vi "LVDeleteFile_Item_OnCommand.vi"(10 "Command ID":string, 11 "Object":T1) -> ()   [LabVIEW 2018]
uses:
  <resource>/Framework/Providers/API/ItemRef.ctl
panel:
  out "error out":errorcluster
  in  "error in":errorcluster
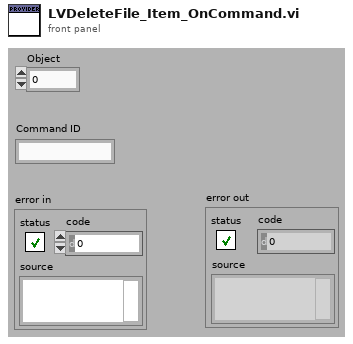
[diagram p1: front panel]
types:
  T1 = typedef "ItemRef.ctl" = u64
  T2 = enum16{"Left Button", "Center Button", "Right Button", "Window Close"}
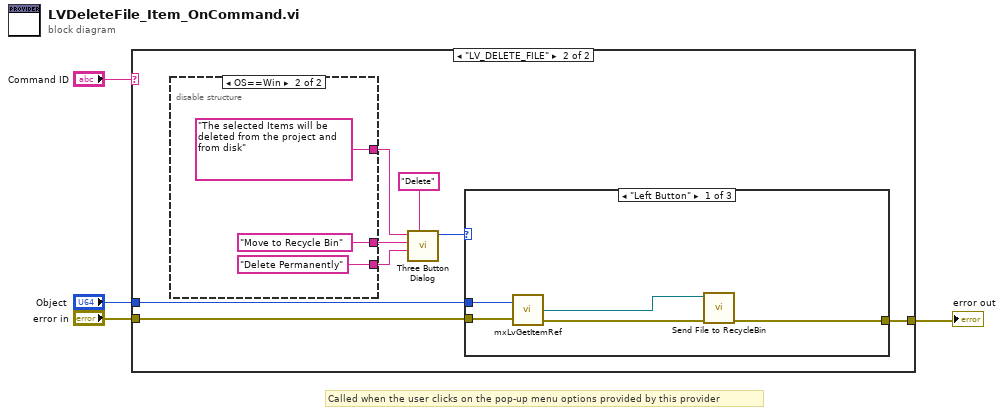
[diagram p0: block diagram]
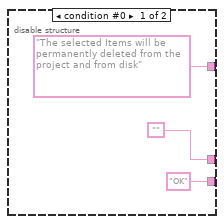
[diagram p3: hidden frame]
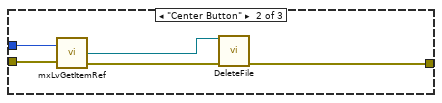
[diagram p4: hidden frame]
diagram:
  # "Called when the user clicks on the pop-up menu options provided by this provider"
  n1 = case shown="\"LV_DELETE_FILE\"" "Command ID" {
    tunnel: "error in" -> [w5 w13]
    tunnel: [w5 w12] -> w2
    tunnel: "Object" -> [_ w11]
    frame Default {
    }
    frame "LV_DELETE_FILE" {
      n2 = disable-structure shown="OS==Win" {
        disable-tunnel: ["The selected Items will be permanently deleted from the project and from disk" ("message") "The selected Items will be deleted from the project and from disk" ("message")] -> w10
        disable-tunnel: ["" "Move to Recycle Bin" ("message")] -> w8
        disable-tunnel: ["OK" ("message") "Delete Permanently" ("message")] -> w7
        frame condition #0 {
        }
        frame condition #1 (active) {
        }
      }
      n3 = call <vilib>:"Three Button Dialog.vi"("Window Title (\"\")"="Delete" ("Window Title (\"\")"), "Center Button Text (\"No\")"=w7, "Left Button Text (\"Yes\")"=w8, "message"=w10) -> ("Which Button?"=w9:T2)  [unwired: 7 in]
      n4 = case shown="\"Left Button\"" w9 {
        tunnel: w11 -> [w24 w29 _]
        tunnel: w13 -> [w23 w28 w30]
        tunnel: [w20 w27 w30] -> w12
        frame "Left Button" {
          n5 = call <resource>:"mxLvGetItemRef.vi"("Item"=w24, "error in"=w23) -> ("Item Refnum"=w22:refnum<vi>, "error out"=w21:errorcluster)  [unwired: 1 out]
          n6 = call "Send File to RecycleBin.vi"("error in"=w21, "Item Refnum"=w22) -> ("error out"=w20:errorcluster)  [unwired: 9 in]
        }
        frame "Center Button" {
          n7 = call <resource>:"mxLvGetItemRef.vi"("Item"=w29, "error in"=w28) -> ("Item Refnum"=w25:refnum<vi>, "error out"=w26:errorcluster)  [unwired: 1 out]
          n8 = call "DeleteFile.vi"("Item Refnum"=w25, "error in"=w26) -> ("error out"=w27:errorcluster)  [unwired: 13 in]
        }
        frame Default {
        }
      }
    }
  }
  "error out" <- w2
